vi "Close.vi"(8 "error in (no error)":errorcluster, 11 "Endpoint in":refnum<class "Endpoint.lvclass">) -> (0 "error out":errorcluster)   [LabVIEW 2020, in "Stream-Simple-Msg.lvlib" / "Endpoint.lvclass"]
uses:
  Endpoint.lvclass
  Endpoint.lvclass/Endpoint.ctl
  <vilib>/IlluminatedG/lv-stream/stream/Stream.lvclass
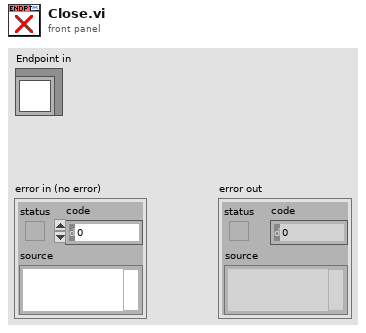
[diagram p1: front panel]
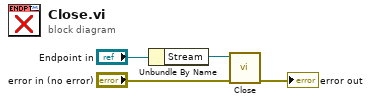
[diagram p0: block diagram]
diagram:
  n1 = Unbundle By Name("Endpoint in") -> ("Stream"=w3:refnum<class "Stream.lvclass">)
  n2 = call-dynamic "Close.vi"("error in (no error)"="error in (no error)", "Stream in"=w3) -> ("error out"=→"error out":errorcluster)  [unwired: 8 in, 1 out]
